vi "ROI grp-Case-Make group visible.vi"(8 "error in (no error)":errorcluster, 10 "Visibility?":bool=TRUE) -> (0 "error out":errorcluster)   [LabVIEW 2020]
uses:
  Globals/gl_ROI grp window globals.vi
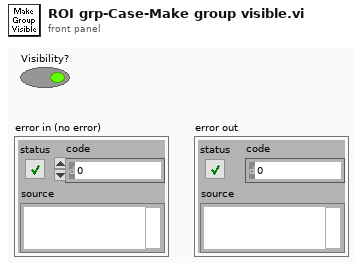
[diagram p1: front panel]
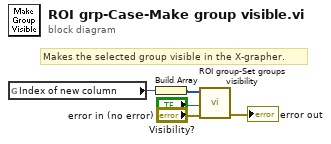
[diagram p0: block diagram]
diagram:
  # "Makes the selected group visible in the X-grapher."
  n1 = global read "gl_ROI grp window globals.vi" "Index of new column"() -> (w4:i32)
  n2 = Build Array(w4) -> (w3:i32[])
  n3 = call "ROI group-Set groups visibility.vi"("error in (no error)"="error in (no error)", "Visibility?"="Visibility?", "Indexes of new groups to make visible"=w3) -> ("error out"=→"error out":errorcluster)  [unwired: 8 in]
